vi "Global Strings.vi"() -> ()   [LabVIEW 2010, in "Agilent 364xA (GPIB,Serial) Custom Device.lvlib"]
uses:
  Agilent 364xA (GPIB,Serial) Custom Device.lvlib
panel:
  in  "FilterTimeoutError":string="FilterTimeoutError"
  in  "ID Query":string="ID Query"
  in  "Update Rate":string="Update Rate"
  in  "Visa Resource Name":string="Visa Resource Name"
  in  "Voltage Limit":string="Voltage Limit"
  in  "Enable OVP":string="Enable OVP"
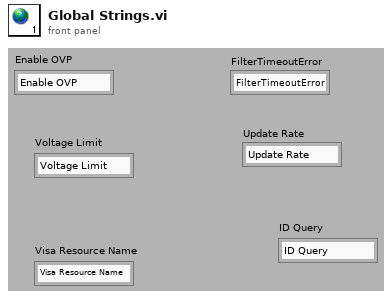
[diagram p1: front panel]
diagram:
